vi "Close Audio File.vi"(8 "error in (no error)":errorcluster, 11 "Audio File Refnum In":T1) -> (0 "error out":errorcluster)   [LabVIEW 2020, in "G-Audio.lvlib"]
doc: "Close an audio file, and clean up the relevant decoder.\n\nThis node runs normally even if an error occurred before this node runs."
uses:
  G-Audio.lvlib
  Controls/Audio File Refnum.ctl
  <vilib>/Utility/error.llb/Error Cluster From Error Code.vi
  lib/g_audio_32.dll
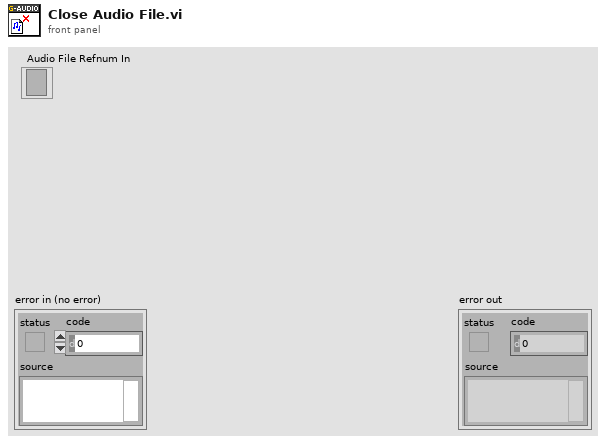
[diagram p1: front panel]
types:
  T1 = typedef "G-Audio.lvlib/Audio File Refnum.ctl" = refnum<file>
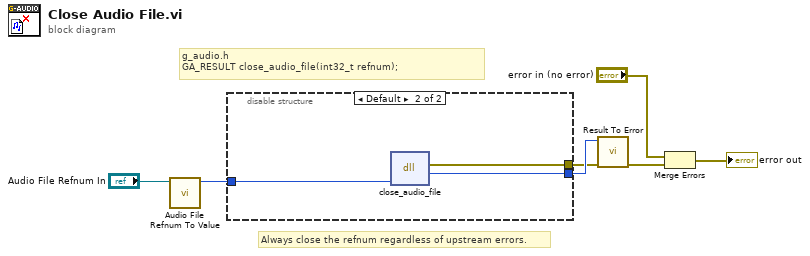
[diagram p0: block diagram]
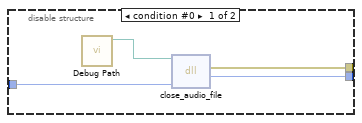
[diagram p2: hidden frame]
diagram:
  # "g_audio.h\nGA_RESULT close_audio_file(int32_t refnum);"
  # "Always close the refnum regardless of upstream errors."
  n1 = call "Audio File Refnum To Value.vi"("Audio File Refnum"="Audio File Refnum In") -> ("Refnum Value"=w7:i32)  [unwired: 10 in]
  n2 = disable-structure shown="Default" {
    disable-tunnel: w7 -> [w11 w14]
    disable-tunnel: [w10 w13] -> w3
    disable-tunnel: [w9 w12] -> w4
    frame condition #0 {
      n3 = call "Debug Path.vi"() -> ("Debug Path"=w8:path)  [unwired: 11 in]
      n4 = dll-call lib="?" fn="close_audio_file"(path in=w8, "refnum"=w11) -> (error out=w10:errorcluster, "result"=w9:i32)  [unwired: 3 in, 1 out]
    }
    frame condition #1 (active) {
      n5 = dll-call lib="C:/github/dataflowg/g-audio/src/LabVIEW/G-Audio/lib/g_audio_*.*" fn="close_audio_file"("refnum"=w14) -> (error out=w13:errorcluster, "result"=w12:i32)  [unwired: 4 in, 1 out]
    }
  }
  n6 = call "Result To Error.vi"("error in (no error)"=w3, "Result Code"=w4) -> ("error out"=w2:errorcluster)  [unwired: 9 in]
  n7 = Merge Errors("error in (no error)", w2) -> (→"error out":errorcluster)
